vi "Release MDPtrQ in Map.vi"(6 "free cache?":bool, 8 "error in (no error)":errorcluster, 11 "MDPtrQ":T1) -> (0 "error out":errorcluster)   [LabVIEW 2017, in "MDPtr.lvlib" / "MDPtrMgr.lvclass"]
uses:
  MDPtrMgr.lvclass
  Factory/Def-MDPtrQ.ctl
  MDPtr TypeDef/MDPtr DataFrame-Memory.ctl
  MDPtr TypeDef/MDPtr DataFrame-Common.ctl
  <vilib>/Utility/Data Type/Type Definitions/Data Type.ctl
  MDPtr.lvlib
  <vilib>/Utility/Data Type/NI_Data Type.lvlib
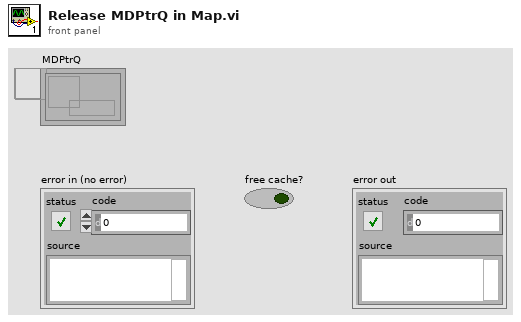
[diagram p1: front panel]
types:
  T1 = typedef "MDPtr.lvlib/MDPtrMgr.lvclass/Def-MDPtrQ.ctl" = refnum<queue>
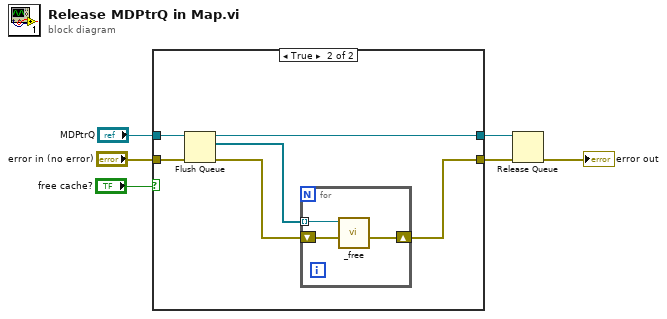
[diagram p0: block diagram]
diagram:
  n1 = case shown="True" "free cache?" {
    tunnel: [w7 w12] -> w6
    tunnel: [w8 w11] -> w5
    tunnel: "MDPtrQ" -> [w8 w10]
    tunnel: "error in (no error)" -> [w7 w9]
    frame False {
    }
    frame True {
      n2 = Flush Queue(queue=w10, error in (no error)=w9) -> (queue out=w11:T1, remaining elements=w14:refnum<data-value>[], error out=w13:errorcluster)
      n3 = for {
        tunnel: w14 -> [w15] mode=indexing
        shift-right: [w16] -> w12
        shift-left: w13 -> [w17]
        n4 = call "_free.vi"("error in (no error)"=w17, "MDPtr DVR"=w15) -> ("error out"=w16:errorcluster)  [unwired: 8 in]
      }
    }
  }
  n5 = Release Queue(queue=w5, error in (no error)=w6) -> (error out=→"error out":errorcluster)  [unwired: 1 in, 2 out]
